vi "Optical Flow Feature Tracking.vi"() -> ()   [LabVIEW 2014]
doc: "This example shows how to use the Lucas Kanade Pyramid motion estimation VI to track features in a sequence of images in NI Vision. The VI reads the frames from an AVI file and tracks user specified features in the image from frame to frame."
uses:
  <vilib>/vision/NI_Vision_Development_Module.lvlib
panel:
  in  "Delay (s.)":dbl(slide)=0.25 scale=0.0..1.5
  out "Image":T1(plugin-control)
  out "Progress Bar":i32(slide) max=63 scale=0.0..63.0
  in  "Stop":bool
  # "Overview: Demonstrate the use of the Optical Flow tracking algorithm of Vision Development Module.\nRequirements: Vision Development Module\nInstructions: Run the VI."
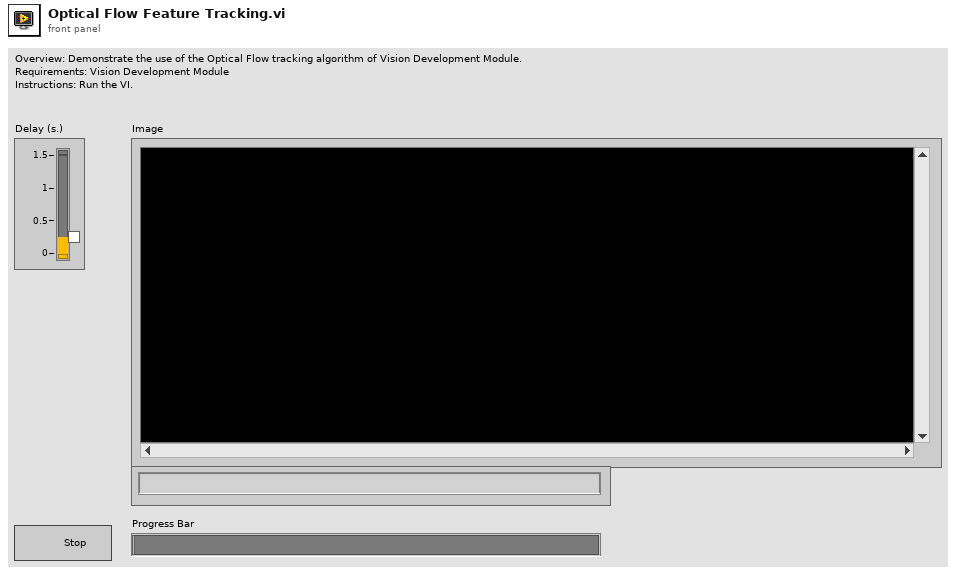
[diagram p1: front panel]
types:
  T1 = typedef "IMAQ Image.ctl" = refnum<image>
  T2 = cluster{"Level":i32, "Max. Iterations":i32, "Window Size":i32, "Displacement Threshold":dbl}
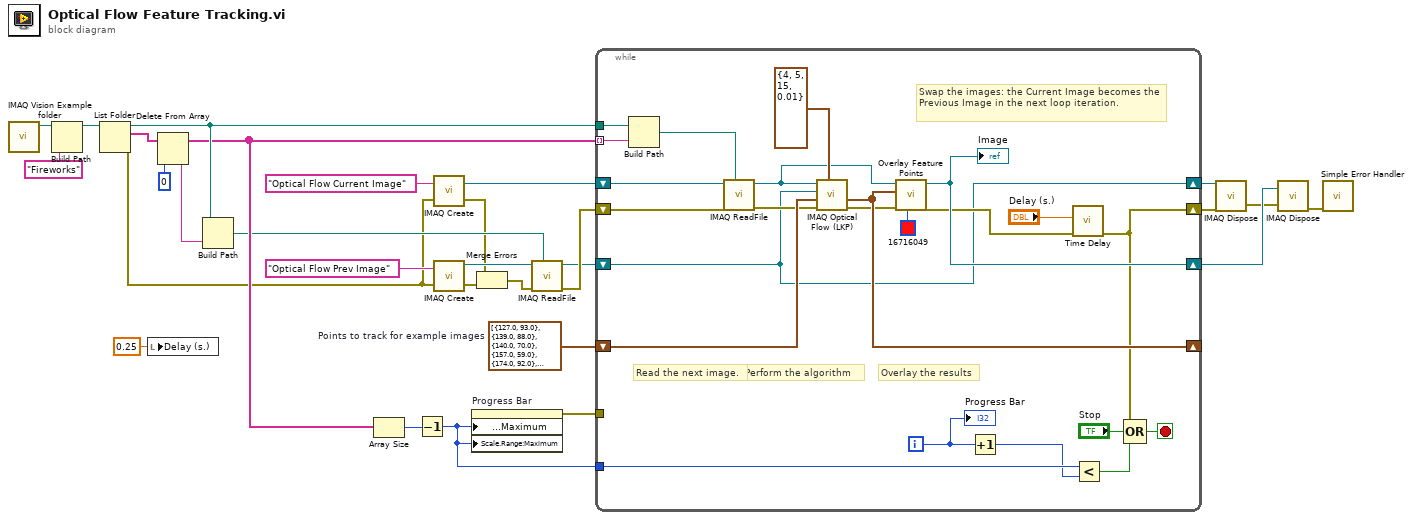
[diagram p0: block diagram]
diagram:
  w13 = cluster{"X":sgl, "Y":sgl}[] [{"X"=127.0, "Y"=93.0}, {"X"=139.0, "Y"=88.0}, {"X"=140.0, "Y"=70.0}, {"X"=157.0, "Y"=59.0}, {"X"=174.0, "Y"=92.0}, {"X"=191.0, "Y"=143.0}, {"X"=215.0, "Y"=53.0}, {"X"=145.0, "Y"=165.0}, {"X"=166.0, "Y"=110.0}]  # Points to track for example images
  n1 = call "IMAQ Vision Example folder.vi"() -> ("Example Image Path"=w3:path)  [unwired: 11 in]
  n2 = Build Path(base path=w3, name or relative path="Fireworks") -> (appended path=w23:path)
  n3 = List Folder(path=w23) -> (path out=w22:path, filenames=w16:string[], error out=w10:errorcluster)  [unwired: 1 in, 3 out]
  n4 = local write "Delay (s.)"(0.25 ("Delay (s)")) -> ()
  n5 = Delete From Array(array=w16, index=0) -> (deleted portion=w24:string, array with subset deleted=w20:string[])  [unwired: 1 in]
  n6 = Build Path(base path=w22, name or relative path=w24) -> (appended path=w18:path)
  n7 = Array Size(array=w20) -> (size(s)=w21:i32)
  n8 = Decrement(x=w21) -> (x-1=w2:i32)
  n9 = call "IMAQ Create"("Image Name"="Optical Flow Current Image", "error in (no error)"=w10) -> ("New Image"=w28:T1, "error out"=w9:errorcluster)  [unwired: 2 in, 1 out]
  n10 = call "IMAQ Create"("Image Name"="Optical Flow Prev Image", "error in (no error)"=w10) -> ("New Image"=w17:T1, "error out"=w8:errorcluster)  [unwired: 2 in, 1 out]
  n11 = property on="Progress Bar" class="Slide (strict)"("Data Entry Limits:Maximum"=w2, "Scale.Range:Maximum"=w2) -> (error out=w27:errorcluster)  [unwired: 2 in, 1 out]
  n12 = Merge Errors(w9, w8) -> (w7:errorcluster)
  n13 = call "IMAQ ReadFile"("File Path"=w18, "error in (no error)"=w7, "Image"=w17) -> ("error out"=w19:errorcluster, "Image Out"=w12:T1)  [unwired: 2 in, 5 out]
  n14 = while {
    tunnel: w2 -> [w49]
    tunnel: w27 -> [_]
    shift-right: [w48] -> w14
    shift-left: w12 -> [w32]
    shift-right: [w46] -> _
    shift-left: w13 -> [w47]
    shift-right: [w42] -> w11
    shift-left: w19 -> [w52]
    tunnel: w22 -> [w44]
    tunnel: w20 -> [w34] mode=indexing
    shift-right: [w32] -> w15
    shift-left: w28 -> [w45]
    i -> [w33]
    stop <- w31 stop-if-true
    # "Swap the images: the Current Image becomes the Previous Image in the next loop iteration."
    # "Overlay the results"
    # "Read the next image."
    # "Perform the algorithm"
    n15 = Build Path(base path=w44, name or relative path=w34) -> (appended path=w35:path)
    n16 = call "IMAQ ReadFile"("File Path"=w35, "error in (no error)"=w52, "Image"=w45) -> ("error out"=w39:errorcluster, "Image Out"=w36:T1)  [unwired: 2 in, 5 out]
    n17 = call "IMAQ Optical Flow (LKP)"("Options"=T2 {"Level"=4, "Max. Iterations"=5, "Window Size"=15, "Displacement Threshold"=0.01}, "error in (no error)"=w39, "Feature Points In"=w47, "Previous Frame"=w32, "Current Frame"=w36) -> ("error out"=w38:errorcluster, "Feature Points Out"=w46:cluster{"X":sgl, "Y":sgl}[])  [unwired: 1 in, 4 out]
    n18 = call "Overlay Feature Points.vi"("Color"=u32 16716049, "error in"=w38, "Feature Points"=w46, "Image"=w36) -> ("error out"=w40:errorcluster, "Image Out"=w48:T1)  [unwired: 2 in, 4 out]
    "Image" <- w48
    n19 = Increment(x=w33) -> (x+1=w43:i32)
    n20 = call "Time Delay"("error in (no error)"=w40, "Delay Time (s)"="Delay (s.)") -> ("error out"=w42:errorcluster)  [unwired: 9 in]
    n21 = Less?(x=w49, y=w43) -> (x < y?=w51:bool)
    n22 = Compound Arithmetic op=OR(w42, "Stop", w51) -> (w31:bool)
    "Progress Bar" <- w33
  }
  n23 = call "IMAQ Dispose"("Image"=w15, "error in (no error)"=w11) -> ("error out"=w5:errorcluster)  [unwired: 1 in, 3 out]
  n24 = call "IMAQ Dispose"("Image"=w14, "error in (no error)"=w5) -> ("error out"=w4:errorcluster)  [unwired: 1 in, 3 out]
  n25 = call <vilib>:"Simple Error Handler.vi"("error in (no error)"=w4) -> ()  [unwired: 1 in, 8 out]
